vi "Teleop.vi"(10 "Match Info":T1={"Autonomous Elapsed Seconds"=0.0, "TeleOp Elapsed Seconds"=0.0, "Disabled Elapsed Seconds"=0.0, "Visited Autonomous"=FALSE, "Visited TeleOp"=FALSE, "Visited Disabled"=FALSE, "Autonomous Settings"={"Autonomous Style"=enum."Independent", "VI Refnum"=refnum}}, 11 "Call Context":T2) -> ()   [LabVIEW 2015]
doc: "This VI is called for each TeleOp packet received from the DS where the robot is not disabled. It is often used to read from the joysticks and update I/O or to update setpoints for timed control loops. It should complete and return within 20 milliseconds or it may miss DS packets."
uses:
  <vilib>/Rock Robotics/WPI/DriverStation/WPI_DriverStationDerivedRobotMode.ctl
  <vilib>/Rock Robotics/WPI/DriverStation/WPI_DriverStationMatch Info.ctl
  Robot Global Data.vi
  <vilib>/Rock Robotics/Network Tables/SD Write Number.vi
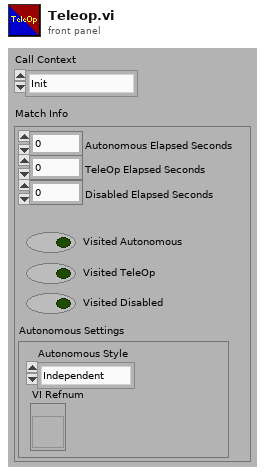
[diagram p1: front panel]
types:
  T1 = typedef "WPI_DriverStationMatch Info.ctl" = cluster{"Autonomous Elapsed Seconds":dbl, "TeleOp Elapsed Seconds":dbl, "Disabled Elapsed Seconds":dbl, "Visited Autonomous":bool, "Visited TeleOp":bool, "Visited Disabled":bool, "Autonomous Settings":cluster{"Autonomous Style":enum16{"Iterative", "Independent"}, "VI Refnum":refnum<vi>}}
  T2 = typedef "WPI_DriverStationDerivedRobotMode.ctl" = enum16{"Init", "Execute", "Stop"}
  T3 = typedef "WPI_RobotDriveDevRef.ctl" = cluster{"DevStatus":errorcluster, "Motors[]":T4[], "Square Inputs":bool, "Max Output":dbl}
  T4 = typedef "WPI_MotorControlDeviceRef.ctl" = cluster{"DeviceStatus":errorcluster, "Type":T5, "PWM":cluster{"PWM Channel":T6, "DeadBand":T7}, "CAN":cluster{"Device Number":u8, "Control Mode":T8, "Semaphore":T9, "Max Vout":dbl, "TalonSRX Control Mode":T10}, "Invert":bool}
  T5 = typedef "WPI_MotorControlType.ctl" = enum16{"PWM", "CAN", "CANTalonSRX"}
  T6 = typedef "FPGA_DIOPWMChannel.ctl" = enum8{"PWM 0", "PWM 1", "PWM 2", "PWM 3", "PWM 4", "PWM 5", "PWM 6", "PWM 7", "PWM 8", "PWM 9", "PWM MXP 0", "PWM MXP 1", "PWM MXP 2", "PWM MXP 3", "PWM MXP 4", "PWM MXP 5", "PWM MXP 6", "PWM MXP 7", "PWM MXP 8", "PWM MXP 9", "Invalid"}
  T7 = typedef "WPI_PWMDeadband.ctl" = cluster{"Name":string, "maxPositivePwm":i32, "minPositivePwm":i32, "centerPwm":i32, "maxNegativePwm":i32, "minNegativePwm":i32, "angularRange":u16}
  T8 = typedef "WPI_CANJaguar_ControlMode.ctl" = enum8{"Percent VBus", "Current", "Speed", "Position", "Voltage"}
  T9 = typedef "Semaphore RefNum" = refnum<k1>
  T10 = typedef "WPI_CANTalonSRX_APIControlMode.ctl" = enum8{"Percent VBus", "Speed", "Position", "Slave", "Unchanged / Invalid", "Voltage Compensation", "Current", "Motion Profile"}
  T11 = typedef "WPI_CANTalonSRX_GlobalStatus.ctl" = cluster{"Applied Throttle":dbl, "Module Enabled":bool, "CAN Error":errorcluster, "Closed Loop Error":dbl, "Forward Limit Switch Closed":bool, "Reverse Limit Switch Closed":bool, "Sensor Position":dbl, "Sensor Velocity":dbl, "Current":dbl, "Sticky Fault - Over Temp":bool, "Sticky Fault - Under Voltage":bool, "Sticky Fault - Forward Limit":bool, "Sticky Fault - Reverse Limit":bool, "Sticky Fault - Forward Soft Limit":bool, "Sticky Fault - Reverse Soft Limit":bool, "Brake is Enabled":bool, "Encoder Position":dbl, "Encoder Velocity":dbl, "Encoder Index Count":dbl, "Encoder A Pin State":bool, "Encoder B Pin State":bool, "Encoder Index Pin State":bool, "Analog In":dbl, "Analog In Velocity":dbl, "Temperature (C)":dbl, "Battery Voltage":dbl, "Control 5 Is Supported":bool, "Current Profile Slot Select":dbl, "Pos Div 8":bool, "Vel Div 4":bool, "Pulse Width Position":i32, "Pulse Width Velocity":i32, "Pulse Width Rise To Rise (us)":i32, "Pulse Width Rise To Fall (us)":i32, "Mot Prof Active Is Under Run":bool, "Mot Prof Active Has Under Run":bool, "Mot Prof Active Is Last":bool, "Mot Prof Active Velocity Only":bool, "Mot Prof Active Is Valid":bool, "Mot Prof Buffer Is Full":bool, "Mot Prof Active Profile Slot Select":i32, "Mot Prof NextID":i32, "Mot Prof Count":i32, "Mot Prof Active Velocity":dbl, "Mot Prof Active Position":dbl, "Mot Prof Output Enable":i32}
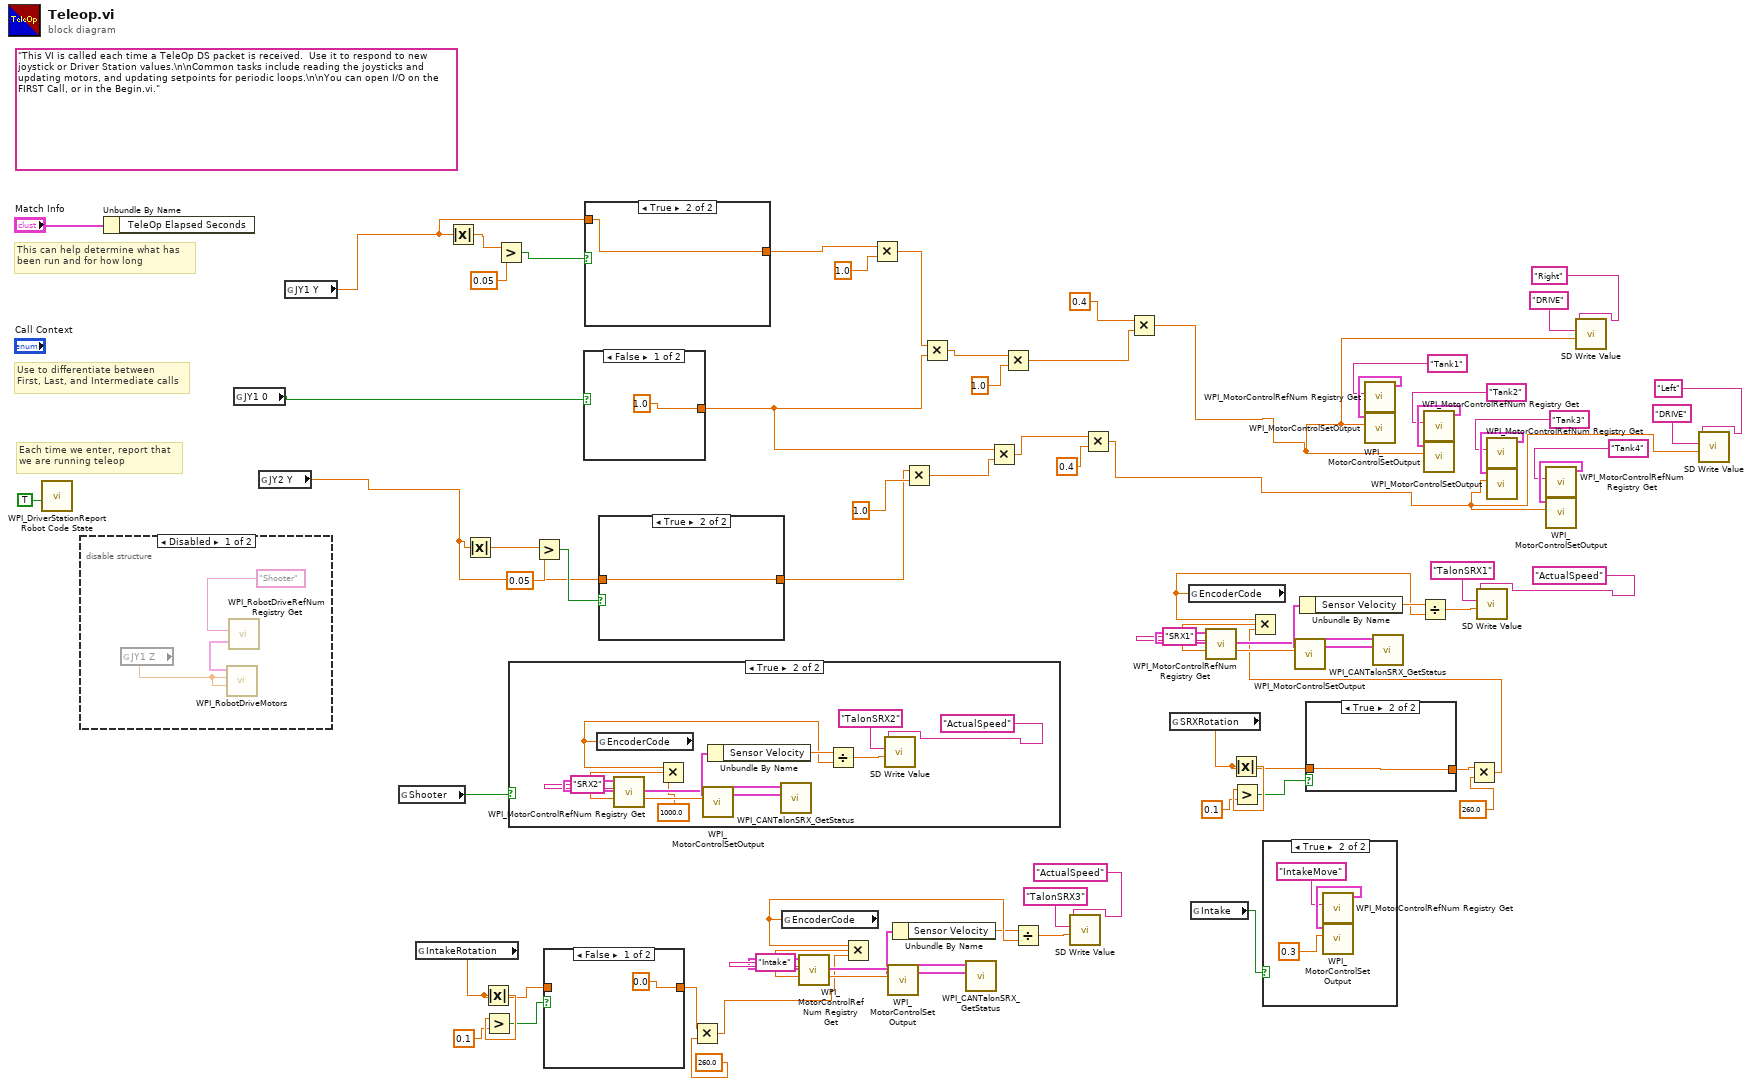
[diagram p0: block diagram]
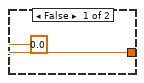
[diagram p4: hidden frame]
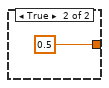
[diagram p7: hidden frame]
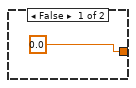
[diagram p8: hidden frame]
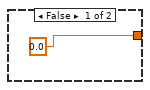
[diagram p9: hidden frame]
diagram:
  (unwired) "This VI is called each time a TeleOp DS packet is received.  Use it to respond to new joystick or Driver Station values.\n\nCommon tasks include reading the joysticks and updating motors, and updating setpoints for periodic loops.\n\nYou can open I/O on the FIRST Call, or in the Begin.vi."
  # "Each time we enter, report that\nwe are running teleop"
  # "Use to differentiate between\nFirst, Last, and Intermediate calls"
  # "This can help determine what has\nbeen run and for how long"
  n1 = call <vilib>:"WPI_DriverStationReport Robot Code State.vi"("TeleOp"=TRUE ("Autonomous")) -> ()  [unwired: 10 in, 1 out]
  n2 = disable-structure shown="Disabled" {
    frame Disabled {
      n3 = global read "Robot Global Data.vi" "JY1 Z"() -> (w75:dbl)
      n4 = call <vilib>:"WPI_RobotDriveRefNum Registry Get.vi"("refnum name"="Shooter") -> ("RobotDriveDevRef"=w76:T3)  [unwired: 1 in, 9 out]
      n5 = call <vilib>:"WPI_RobotDriveMotors.vi"("RightSpeed"=w75, "LeftSpeed"=w75, "RobotDriveDevRef"=w76) -> ()  [unwired: 6 in, 3 out]
    }
    frame Enabled {
    }
  }
  n6 = Unbundle By Name("Match Info") -> ()  [unwired: 1 out]
  n7 = global read "Robot Global Data.vi" "JY1 0"() -> (w51:bool)
  n8 = global read "Robot Global Data.vi" "JY2 Y"() -> (w52:dbl)
  n9 = global read "Robot Global Data.vi" "JY1 Y"() -> (w53:dbl)
  n10 = global read "Robot Global Data.vi" "Shooter"() -> (w40:bool)
  n11 = global read "Robot Global Data.vi" "IntakeRotation"() -> (w5:dbl)
  n12 = Absolute Value(x=w53) -> (abs(x)=w57:dbl)
  n13 = Absolute Value(x=w52) -> (abs(x)=w56:dbl)
  n14 = Absolute Value(x=w5) -> (abs(x)=w10:dbl)
  n15 = Greater?(x=w10, y=0.1) -> (0:w8:bool)
  n16 = Greater?(x=w57, y=0.05) -> (0:w72:bool)
  n17 = case shown="True" w40 {
    frame False {
    }
    frame True {
      n18 = global read "Robot Global Data.vi" "EncoderCode"() -> (w84:dbl)
      n19 = call <vilib>:"WPI_MotorControlRefNum Registry Get.vi"("refnum name"="SRX2") -> ("MotorControlDevRef"=w82:T4)  [unwired: 9 in, 1 out]
      n20 = Multiply(x=w84, y=1000.0) -> (x*y=w85:dbl)
      n21 = call <vilib>:"WPI_MotorControlSetOutput.vi"("Output"=w85, "MotorControlDevRef"=w82) -> ("MotorControlDevRef"=w88:T4)  [unwired: 7 in, 2 out]
      n22 = call <vilib>:"WPI_CANTalonSRX_GetStatus.vi"("CAN Talon SRX Ref"=w88) -> ("Talon SRX Status"=w87:T11)  [unwired: 8 in, 2 out]
      n23 = Unbundle By Name(w87) -> ("Sensor Velocity"=w86:dbl)
      n24 = Divide(x=w86, y=w84) -> (x/y=w81:dbl)
      n25 = call-poly <vilib>:"SD Write Value.vi"("Numeric"=w81, "Table Prefix"="TalonSRX2", "Name"="ActualSpeed") -> ()  [unwired: 7 in, 2 out]
    }
  }
  n26 = Greater?(x=w56, y=0.05) -> (0:w70:bool)
  n27 = case shown="False" w8 {
    tunnel: w5 -> [_ w90]
    tunnel: [0.0 w90] -> w7
    frame False {
    }
    frame True {
    }
  }
  n28 = case shown="False" w51 {
    tunnel: [1.0 0.5] -> w63
    frame False {
    }
    frame True {
    }
  }
  n29 = case shown="True" w72 {
    tunnel: [0.0 w94] -> w66
    tunnel: w53 -> [_ w94]
    frame False {
    }
    frame True {
    }
  }
  n30 = case shown="True" w70 {
    tunnel: [0.0 w96] -> w65
    tunnel: w52 -> [_ _]
    tunnel: w52 -> [_ w96]
    frame False {
    }
    frame True {
    }
  }
  n31 = Multiply(x=w7, y=260.0) -> (x*y=w6:dbl)
  n32 = global read "Robot Global Data.vi" "EncoderCode"() -> (w16:dbl)
  n33 = call <vilib>:"WPI_MotorControlRefNum Registry Get.vi"("refnum name"="Intake") -> ("MotorControlDevRef"=w18:T4)  [unwired: 9 in, 1 out]
  n34 = Multiply(x=w16, y=w6) -> (x*y=w15:dbl)
  n35 = Multiply(x=w66, y=1.0) -> (x*y=w64:dbl)
  n36 = call <vilib>:"WPI_MotorControlSetOutput.vi"("Output"=w15, "MotorControlDevRef"=w18) -> ("MotorControlDevRef"=w12:T4)  [unwired: 7 in, 2 out]
  n37 = Multiply(x=w65, y=1.0) -> (x*y=w62:dbl)
  n38 = Multiply(x=w64, y=w63) -> (x*y=w61:dbl)
  n39 = call <vilib>:"WPI_CANTalonSRX_GetStatus.vi"("CAN Talon SRX Ref"=w12) -> ("Talon SRX Status"=w13:T11)  [unwired: 8 in, 2 out]
  n40 = Unbundle By Name(w13) -> ("Sensor Velocity"=w14:dbl)
  n41 = Multiply(x=w63, y=w62) -> (x*y=w58:dbl)
  n42 = Multiply(x=w61, y=1.0) -> (x*y=w54:dbl)
  n43 = Divide(x=w14, y=w16) -> (x/y=w19:dbl)
  n44 = call-poly <vilib>:"SD Write Value.vi"("Numeric"=w19, "Table Prefix"="TalonSRX3", "Name"="ActualSpeed") -> ()  [unwired: 7 in, 2 out]
  n45 = Multiply(x=w58, y=0.4) -> (x*y=w1:dbl)
  n46 = Multiply(x=0.4, y=w54) -> (x*y=w2:dbl)
  n47 = global read "Robot Global Data.vi" "SRXRotation"() -> (w34:dbl)
  n48 = global read "Robot Global Data.vi" "EncoderCode"() -> (w46:dbl)
  n49 = global read "Robot Global Data.vi" "Intake"() -> (w3:bool)
  n50 = call <vilib>:"WPI_MotorControlRefNum Registry Get.vi"("refnum name"="SRX1") -> ("MotorControlDevRef"=w44:T4)  [unwired: 9 in, 1 out]
  n51 = Absolute Value(x=w34) -> (abs(x)=w39:dbl)
  n52 = Greater?(x=w39, y=0.1) -> (0:w38:bool)
  n53 = case shown="True" w3 {
    frame False {
    }
    frame True {
      n54 = call <vilib>:"WPI_MotorControlRefNum Registry Get.vi"("refnum name"="IntakeMove") -> ("MotorControlDevRef"=w99:T4)  [unwired: 9 in, 1 out]
      n55 = call <vilib>:"WPI_MotorControlSetOutput.vi"("Output"=0.3, "MotorControlDevRef"=w99) -> ()  [unwired: 7 in, 3 out]
    }
  }
  n56 = case shown="True" w38 {
    tunnel: [0.0 w101] -> w35
    tunnel: w34 -> [_ w101]
    frame False {
    }
    frame True {
    }
  }
  n57 = call <vilib>:"WPI_MotorControlRefNum Registry Get.vi"("refnum name"="Tank1") -> ("MotorControlDevRef"=w32:T4)  [unwired: 9 in, 1 out]
  n58 = call <vilib>:"WPI_MotorControlSetOutput.vi"("Output"=w2, "MotorControlDevRef"=w32) -> ()  [unwired: 7 in, 3 out]
  n59 = call <vilib>:"WPI_MotorControlRefNum Registry Get.vi"("refnum name"="Tank2") -> ("MotorControlDevRef"=w30:T4)  [unwired: 9 in, 1 out]
  n60 = call <vilib>:"WPI_MotorControlSetOutput.vi"("Output"=w2, "MotorControlDevRef"=w30) -> ()  [unwired: 7 in, 3 out]
  n61 = Multiply(x=w35, y=260.0) -> (x*y=w33:dbl)
  n62 = Multiply(x=w46, y=w33) -> (x*y=w47:dbl)
  n63 = call <vilib>:"WPI_MotorControlSetOutput.vi"("Output"=w47, "MotorControlDevRef"=w44) -> ("MotorControlDevRef"=w50:T4)  [unwired: 7 in, 2 out]
  n64 = call <vilib>:"WPI_CANTalonSRX_GetStatus.vi"("CAN Talon SRX Ref"=w50) -> ("Talon SRX Status"=w49:T11)  [unwired: 8 in, 2 out]
  n65 = Unbundle By Name(w49) -> ("Sensor Velocity"=w48:dbl)
  n66 = Divide(x=w48, y=w46) -> (x/y=w43:dbl)
  n67 = call-poly <vilib>:"SD Write Value.vi"("Numeric"=w43, "Table Prefix"="TalonSRX1", "Name"="ActualSpeed") -> ()  [unwired: 7 in, 2 out]
  n68 = call <vilib>:"WPI_MotorControlRefNum Registry Get.vi"("refnum name"="Tank3") -> ("MotorControlDevRef"=w28:T4)  [unwired: 9 in, 1 out]
  n69 = call <vilib>:"WPI_MotorControlSetOutput.vi"("Output"=w1, "MotorControlDevRef"=w28) -> ()  [unwired: 7 in, 3 out]
  n70 = call <vilib>:"WPI_MotorControlRefNum Registry Get.vi"("refnum name"="Tank4") -> ("MotorControlDevRef"=w26:T4)  [unwired: 9 in, 1 out]
  n71 = call <vilib>:"WPI_MotorControlSetOutput.vi"("Output"=w1, "MotorControlDevRef"=w26) -> ()  [unwired: 7 in, 3 out]
  n72 = call-poly <vilib>:"SD Write Value.vi"("Numeric"=w2, "Table Prefix"="DRIVE", "Name"="Right") -> ()  [unwired: 7 in, 2 out]
  n73 = call-poly <vilib>:"SD Write Value.vi"("Numeric"=w1, "Table Prefix"="DRIVE", "Name"="Left") -> ()  [unwired: 7 in, 2 out]
